vi "Build Transfer.vi"(8 "error in (no error)":errorcluster, 9 "inline?":bool, 10 "Transfer":refnum<class "Transfer.lvclass">, 11 "Buffer Converter in":refnum<class "Buffer Converter.lvclass">) -> (0 "error out":errorcluster, 3 "Buffer Converter out":refnum<class "Buffer Converter.lvclass">)   [LabVIEW 2017, in "DSF Core.lvlib" / "Buffer Converter.lvclass"]
uses:
  Buffer Converter.lvclass
  Transfer/Transfer.lvclass
  Buffer Converter.lvclass/Buffer Converter.ctl
  Transfer/Transfer.lvclass/Transfer.ctl
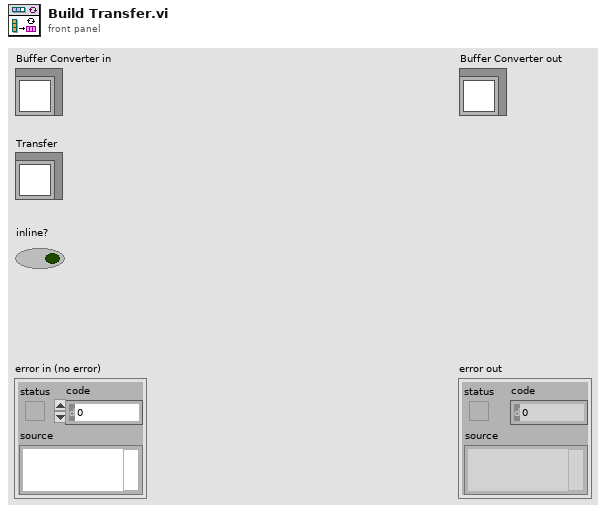
[diagram p1: front panel]
types:
  T1 = typedef "DSF Core.lvlib/Buffer Converter.lvclass/Buffer Conversion Descriptor.ctl" = cluster{"conversions":T2[]}
  T2 = typedef "DSF Core.lvlib/Buffer Converter.lvclass/Conversion.ctl" = cluster{"unconverted descriptor":T3, "converted descriptor":T3, "channel count":u64}
  T3 = typedef "DSF Core.lvlib/Buffer Converter.lvclass/Channel Descriptor.ctl" = cluster{"buffer offset":u64, "data type":T4}
  T4 = typedef "DSF Core.lvlib/DSF Data Type.ctl" = enum8{"Bool", "SGL", "DBL", "I8", "I16", "I32", "I64", "U8", "U16", "U32", "U64"}
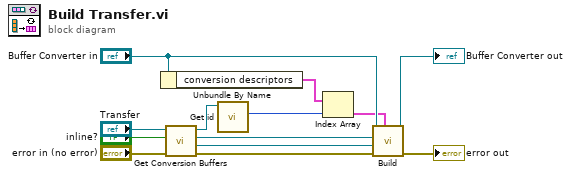
[diagram p0: block diagram]
diagram:
  n1 = Unbundle By Name("Buffer Converter in") -> ("conversion descriptors"=w3:T1[])
  n2 = call "Get Conversion Buffers.vi"("error in (no error)"="error in (no error)", "inline?"="inline?", "Transfer in"="Transfer") -> ("error out"=w9:errorcluster, "converted Buffer"=w7:refnum<class "Buffer.lvclass">, "unconverted Buffer"=w8:refnum<class "Buffer.lvclass">, "Transfer out"=w5:refnum<class "Transfer.lvclass">)  [unwired: 5 in]
  n3 = call "Get id.vi"("Transfer in"=w5) -> ("id"=w2:i32)  [unwired: 9 in, 1 out]
  n4 = Index Array(array=w3, index=w2) -> (element=w1:T1)
  n5 = call-dynamic "Build.vi"("conversion descriptor"=w1, "error in (no error)"=w9, "converted Buffer"=w7, "unconverted Buffer"=w8, "Buffer Converter in"="Buffer Converter in") -> ("error out"=→"error out":errorcluster, "Buffer Converter out"=→"Buffer Converter out":refnum<class "Buffer Converter.lvclass">)  [unwired: 5 in]
